vi "SeCrTS-DD NS Data.vi"(7 "NOT DIS Out":T1, 8 "value":T2, 9 "AI_V_Data P\nAI_C_Data P\nAO_Data P\nDO_Data P\nACC_Data P\nTC Data P\nDrive_A_C \nDrive_A_D\nAI_C_Data S\nDO_Data S":refnum<queue>[](array[refnum]), 11 "DI P\nDI S":refnum<queue>[](array[refnum])) -> ()   [LabVIEW 2022 SP3]
uses:
  Control/SeCrTS-Notifier Ref.ctl
panel:
  out "overflow? 9":bool
  out "overflow? 8":bool
  out "overflow? 7":bool
  out "overflow? 6":bool
  out "overflow? 5":bool
  out "overflow? 4":bool
  out "overflow? 3":bool
  out "overflow? 2":bool
  out "overflow?":bool
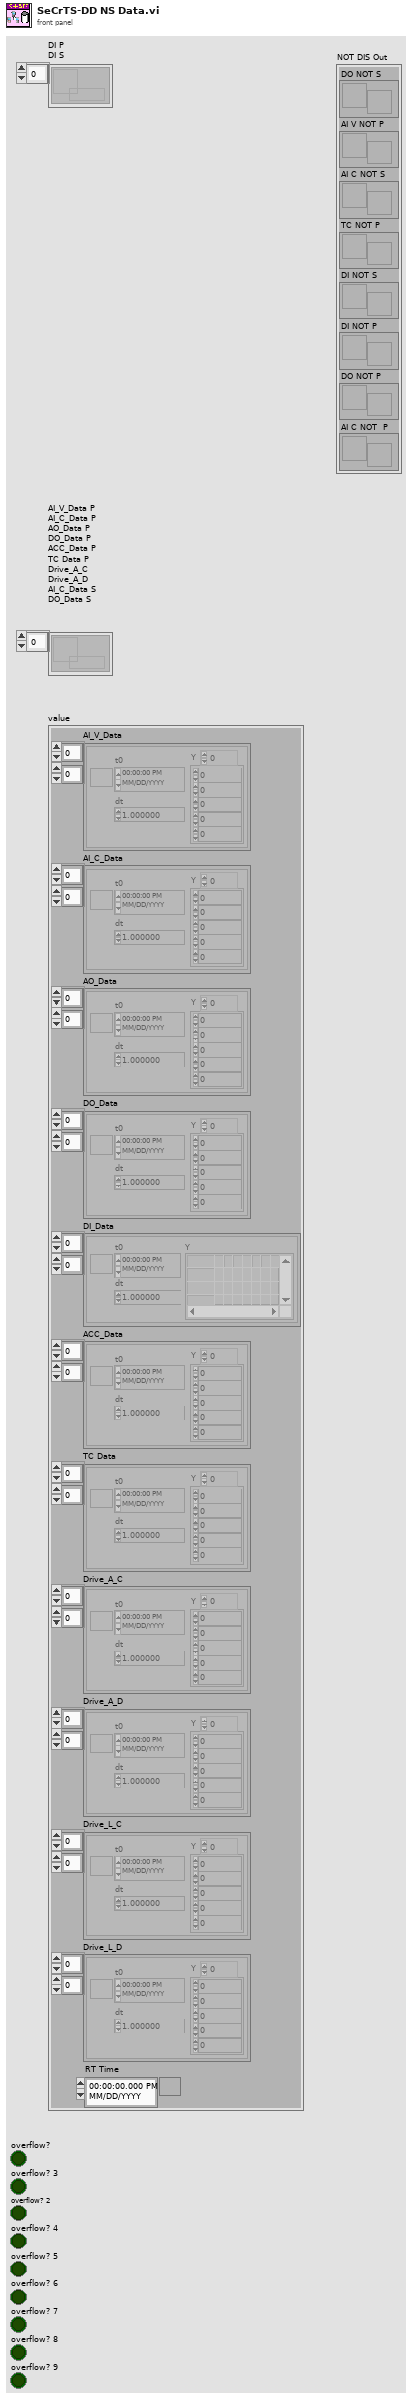
[diagram p1: front panel]
types:
  T1 = typedef "SeCrTS-Notifier Ref.ctl" = cluster{"DO NOT S":refnum<notifier>, "AI V NOT P":refnum<notifier>, "AI C NOT S":refnum<notifier>, "TC NOT P":refnum<notifier>, "DI NOT S":refnum<notifier>, "DI NOT P":refnum<notifier>, "DO NOT P":refnum<notifier>, "AI C NOT  P":refnum<notifier>}
  T2 = cluster{"AI_V_Data":waveform(dbl)[][], "AI_C_Data":waveform(dbl)[][], "AO_Data":waveform(dbl)[][], "DO_Data":waveform(dbl)[][], "DI_Data":digitalwaveform[][], "ACC_Data":waveform(dbl)[][], "TC Data":waveform(dbl)[][], "Drive_A_C":waveform(dbl)[][], "Drive_A_D":waveform(dbl)[][], "Drive_L_C":waveform(dbl)[][], "Drive_L_D":waveform(dbl)[][], "RT Time":timestamp}
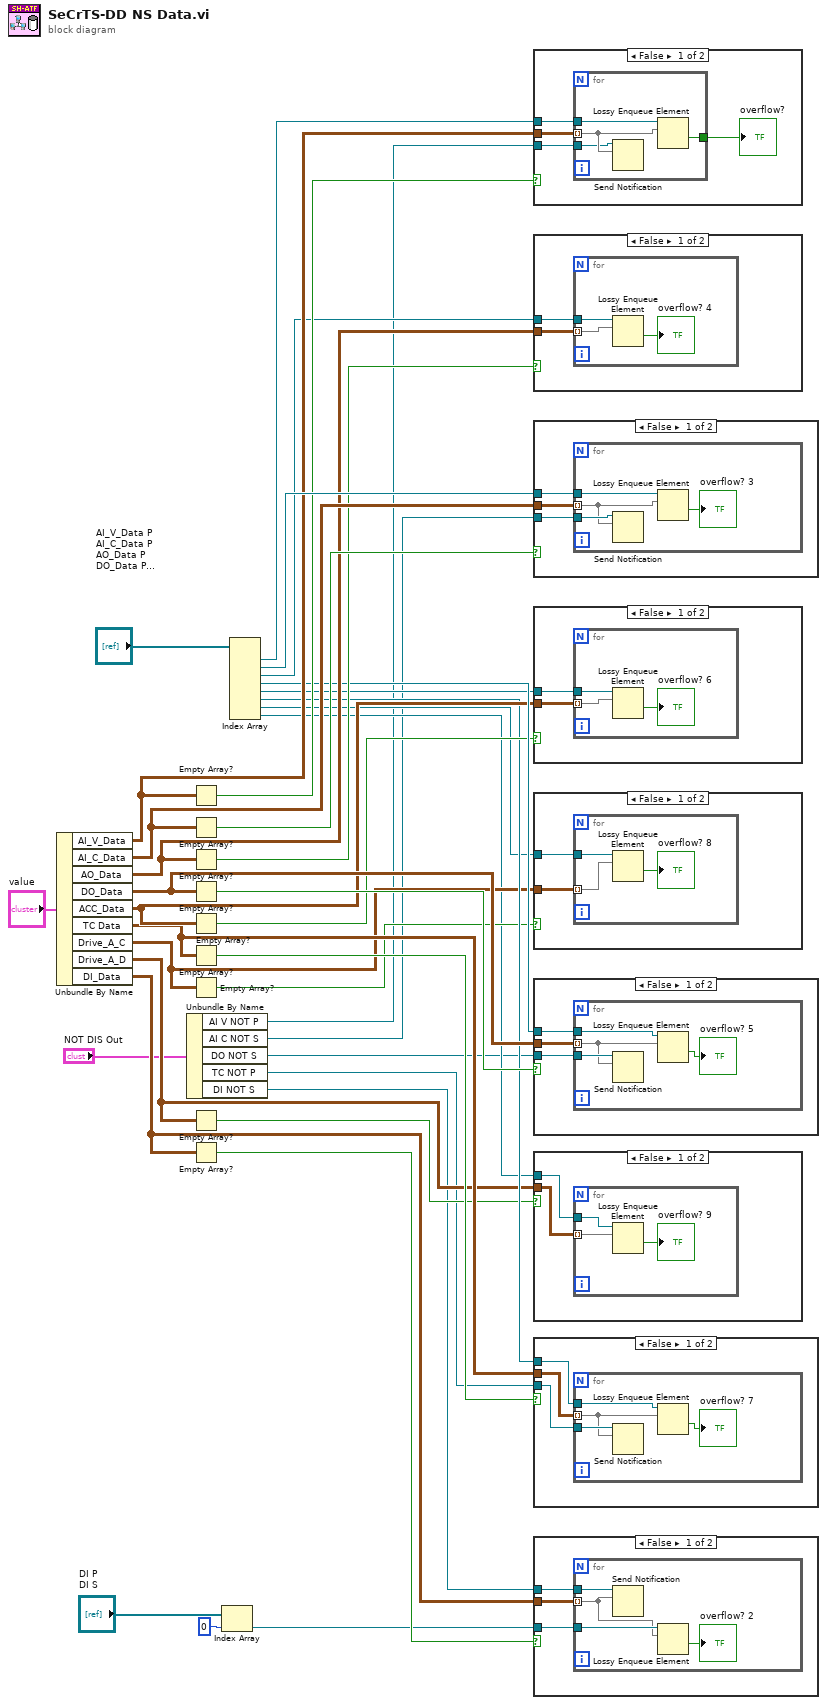
[diagram p0: block diagram]
diagram:
  n1 = Unbundle By Name("value") -> ("AI_V_Data"=w29:waveform(dbl)[][], "AI_C_Data"=w31:waveform(dbl)[][], "AO_Data"=w25:waveform(dbl)[][], "DO_Data"=w22:waveform(dbl)[][], "ACC_Data"=w20:waveform(dbl)[][], "TC Data"=w17:waveform(dbl)[][], "Drive_A_C"=w14:waveform(dbl)[][], "Drive_A_D"=w11:waveform(dbl)[][], "DI_Data"=w33:digitalwaveform[][])
  n2 = Unbundle By Name("NOT DIS Out") -> ("AI V NOT P"=w9:refnum<notifier>, "AI C NOT S"=w8:refnum<notifier>, "DO NOT S"=w7:refnum<notifier>, "TC NOT P"=w6:refnum<notifier>, "DI NOT S"=w5:refnum<notifier>)
  n3 = Empty Array?(array=w29) -> (empty?=w30:bool)
  n4 = Empty Array?(array=w31) -> (empty?=w32:bool)
  n5 = Empty Array?(array=w25) -> (empty?=w27:bool)
  n6 = Empty Array?(array=w22) -> (empty?=w24:bool)
  n7 = Empty Array?(array=w20) -> (empty?=w19:bool)
  n8 = Empty Array?(array=w17) -> (empty?=w16:bool)
  n9 = Empty Array?(array=w14) -> (empty?=w13:bool)
  n10 = Empty Array?(array=w11) -> (empty?=w10:bool)
  n11 = Empty Array?(array=w33) -> (empty?=w34:bool)
  n12 = Index Array(array="DI P\nDI S", index=0) -> (element=w2:refnum<queue>)
  n13 = Index Array(array="AI_V_Data P\nAI_C_Data P\nAO_Data P\nDO_Data P\nACC_Data P\nTC Data P\nDrive_A_C \nDrive_A_D\nAI_C_Data S\nDO_Data S") -> (element #1=w36:refnum<queue>, element #2=w37:refnum<queue>, element #3=w26:refnum<queue>, element #4=w23:refnum<queue>, element #5=w21:refnum<queue>, element #6=w18:refnum<queue>, element #7=w15:refnum<queue>, element #8=w12:refnum<queue>)  [unwired: 8 in]
  n14 = case shown="False" w30 {
    tunnel: w29 -> [w41 _]
    tunnel: w36 -> [w40 _]
    tunnel: w9 -> [w38 _]
    frame False {
      n15 = for {
        tunnel: w41 -> [w43] mode=indexing
        tunnel: w40 -> [w45]
        tunnel: [w44] -> w39
        tunnel: w38 -> [w42]
        n16 = Send Notification(notification=w43, notifier=w42) -> ()  [unwired: 1 in, 2 out]
        n17 = Lossy Enqueue Element(queue=w45, element=w43) -> (overflow?=w44:bool)  [unwired: 1 in, 3 out]
      }
      "overflow?" <- w39
    }
    frame True {
    }
  }
  n18 = case shown="False" w27 {
    tunnel: w25 -> [w47 _]
    tunnel: w26 -> [w46 _]
    frame False {
      n19 = for {
        tunnel: w47 -> [w50] mode=indexing
        tunnel: w46 -> [w49]
        n20 = Lossy Enqueue Element(queue=w49, element=w50) -> (overflow?=→"overflow? 4":bool)  [unwired: 1 in, 3 out]
      }
    }
    frame True {
    }
  }
  n21 = case shown="False" w32 {
    tunnel: w31 -> [w53 _]
    tunnel: w37 -> [w52 _]
    tunnel: w8 -> [w51 _]
    frame False {
      n22 = for {
        tunnel: w53 -> [w54] mode=indexing
        tunnel: w52 -> [w57]
        tunnel: w51 -> [w55]
        n23 = Send Notification(notification=w54, notifier=w55) -> ()  [unwired: 1 in, 2 out]
        n24 = Lossy Enqueue Element(queue=w57, element=w54) -> (overflow?=→"overflow? 3":bool)  [unwired: 1 in, 3 out]
      }
    }
    frame True {
    }
  }
  n25 = case shown="False" w19 {
    tunnel: w20 -> [w59 _]
    tunnel: w21 -> [w58 _]
    frame False {
      n26 = for {
        tunnel: w59 -> [w60] mode=indexing
        tunnel: w58 -> [w62]
        n27 = Lossy Enqueue Element(queue=w62, element=w60) -> (overflow?=→"overflow? 6":bool)  [unwired: 1 in, 3 out]
      }
    }
    frame True {
    }
  }
  n28 = case shown="False" w13 {
    tunnel: w14 -> [w64 _]
    tunnel: w15 -> [w63 _]
    frame False {
      n29 = for {
        tunnel: w64 -> [w65] mode=indexing
        tunnel: w63 -> [w67]
        n30 = Lossy Enqueue Element(queue=w67, element=w65) -> (overflow?=→"overflow? 8":bool)  [unwired: 1 in, 3 out]
      }
    }
    frame True {
    }
  }
  n31 = case shown="False" w24 {
    tunnel: w22 -> [w70 _]
    tunnel: w23 -> [w69 _]
    tunnel: w7 -> [w68 _]
    frame False {
      n32 = for {
        tunnel: w70 -> [w71] mode=indexing
        tunnel: w69 -> [w74]
        tunnel: w68 -> [w72]
        n33 = Send Notification(notification=w71, notifier=w72) -> ()  [unwired: 1 in, 2 out]
        n34 = Lossy Enqueue Element(queue=w74, element=w71) -> (overflow?=→"overflow? 5":bool)  [unwired: 1 in, 3 out]
      }
    }
    frame True {
    }
  }
  n35 = case shown="False" w10 {
    tunnel: w11 -> [w76 _]
    tunnel: w12 -> [w75 _]
    frame False {
      n36 = for {
        tunnel: w76 -> [w77] mode=indexing
        tunnel: w75 -> [w79]
        n37 = Lossy Enqueue Element(queue=w79, element=w77) -> (overflow?=→"overflow? 9":bool)  [unwired: 1 in, 3 out]
      }
    }
    frame True {
    }
  }
  n38 = case shown="False" w16 {
    tunnel: w17 -> [w82 _]
    tunnel: w18 -> [w81 _]
    tunnel: w6 -> [w80 _]
    frame False {
      n39 = for {
        tunnel: w82 -> [w83] mode=indexing
        tunnel: w81 -> [w86]
        tunnel: w80 -> [w84]
        n40 = Send Notification(notification=w83, notifier=w84) -> ()  [unwired: 1 in, 2 out]
        n41 = Lossy Enqueue Element(queue=w86, element=w83) -> (overflow?=→"overflow? 7":bool)  [unwired: 1 in, 3 out]
      }
    }
    frame True {
    }
  }
  n42 = case shown="False" w34 {
    tunnel: w33 -> [w89 _]
    tunnel: w2 -> [w88 _]
    tunnel: w5 -> [w87 _]
    frame False {
      n43 = for {
        tunnel: w89 -> [w90] mode=indexing
        tunnel: w88 -> [w93]
        tunnel: w87 -> [w91]
        n44 = Send Notification(notification=w90, notifier=w91) -> ()  [unwired: 1 in, 2 out]
        n45 = Lossy Enqueue Element(queue=w93, element=w90) -> (overflow?=→"overflow? 2":bool)  [unwired: 1 in, 3 out]
      }
    }
    frame True {
    }
  }
